vi "DB Import Action - Create Chans - Dynamic.vi"(8 "error in (no error)":errorcluster, 10 "selected path":path, 11 "Node Ptr":u64) -> (0 "error out":errorcluster, 2 "selected path out":path caption="selected path", 3 "Node Ptr dup":u64, 5 "Item Ref":T1 format="%.0x")   [LabVIEW 2013]
uses:
  <vilib>/NI Veristand/Custom Device API/Custom Device Item Ref.ctl
  AIT 664 Custom Device.lvlib
  <vilib>/NI Veristand/Custom Device API/Custom Device API.lvlib
panel:
  # "Loading Simulyzer Configuration...\nPlease Wait"
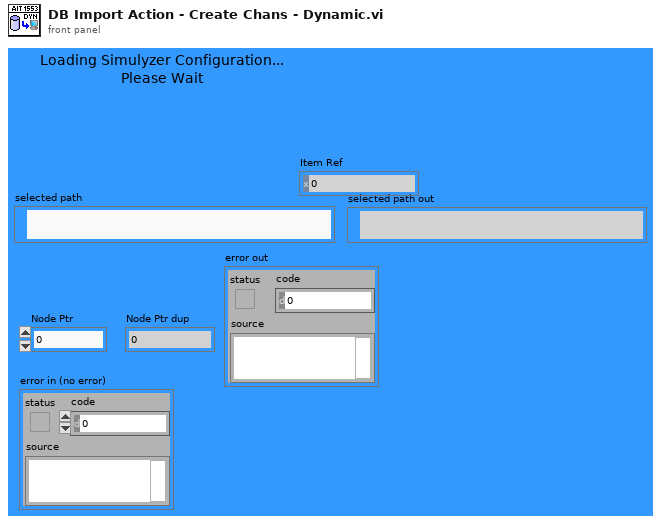
[diagram p1: front panel]
types:
  T1 = typedef "Custom Device API.lvlib/Custom Device Item Ref.ctl" = u64
  T2 = typedef "AIT 664 Custom Device.lvlib/1553_Bus.ctl" = cluster{"Name":string, "Bus_Number":u8, "Bus_Controller":T3, "Bus_Monitor":T7, "RT_Messages":T9[]}
  T3 = typedef "AIT 664 Custom Device.lvlib/1553_Bus_Controller.ctl" = cluster{"BC_Messages":T4[], "Acyclic_Frames":T6[], "Enabled":bool}
  T4 = typedef "AIT 664 Custom Device.lvlib/1553_BC_Message.ctl" = cluster{"Name":string, "Tx-Rx_T-Tx":bool, "RT_Address":u8, "RT_SA_Address":u8, "Parameters":T5[], "Transfer Enabled":bool, "Message Buffer ID":u16, "Default_Message_Buffer_Data":u16[], "Word_Count":u8}
  T5 = typedef "AIT 664 Custom Device.lvlib/1553 Param.ctl" = cluster{"name":string, "firstWord":i32, "startBit":i32, "numberBits":i32, "scaleFactor":dbl, "scaleOffset":dbl, "signed":bool}
  T6 = typedef "AIT 664 Custom Device.lvlib/1553_Acyclic_Frame.ctl" = cluster{"Frame_Index":u8, "Initiate_Xfer":bool}
  T7 = typedef "AIT 664 Custom Device.lvlib/1553_Bus_Monitor.ctl" = cluster{"Name":string, "BM_Messages":T8[], "Address Set Inverted":bool}
  T8 = typedef "AIT 664 Custom Device.lvlib/1553_BM_Message.ctl" = cluster{"RT_Address":u8, "RT_SubAddress":u8, "Tx-Rx_T-Tx":bool, "Parameters":T5[], "Name":string}
  T9 = typedef "AIT 664 Custom Device.lvlib/1553_RT_Message.ctl" = cluster{"RT_Address":u8, "RT_SubAddress":u8, "Tx-Rx_T-Tx":bool, "Parameters":T5[], "Message_Buffer ID":u16, "Default_Message_Buffer_Data":u16[], "Word_Count":u8, "Name":string}
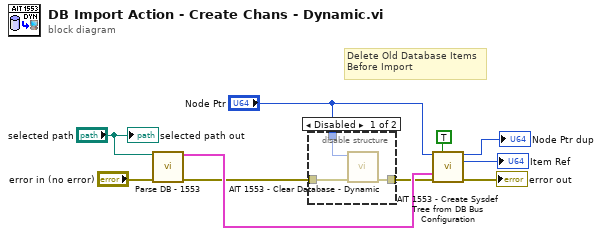
[diagram p0: block diagram]
diagram:
  # "Delete Old Database Items\nBefore Import"
  n1 = call "Parse DB - 1553.vi"("Path in"="selected path", "error in (no error)"="error in (no error)") -> ("Bus"=w5:T2, "error out"=w2:errorcluster)  [unwired: 12 in]
  n2 = disable-structure shown="Disabled" {
    disable-tunnel: [w13 w14] -> w4
    disable-tunnel: "Node Ptr" -> [w12 _]
    disable-tunnel: w2 -> [w11 w14]
    frame Disabled {
      n3 = call "AIT 1553 - Clear Database - Dynamic.vi"("error in (no error)"=w11, "Node Ptr"=w12) -> ("error out"=w13:errorcluster)  [unwired: 9 in]
    }
    frame Enabled {
    }
  }
  n4 = call "AIT 1553 - Create Sysdef Tree from DB Bus Configuration.vi"("Section Ref in"="Node Ptr", "Called From SysDef API (F)"=TRUE, "Bus"=w5, "error in"=w4) -> ("Section Ref out"=→"Node Ptr dup":T1, "Item Ref"=→"Item Ref":T1, "error out"=→"error out":errorcluster)  [unwired: 9 in]
  "selected path out" <- "selected path"
